vi "GetTangent(SubVI).vi"(10 "sn":string) -> (2 "output frame":string)   [LabVIEW 2012]
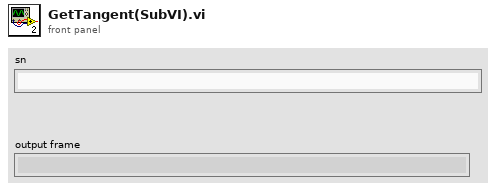
[diagram p1: front panel]
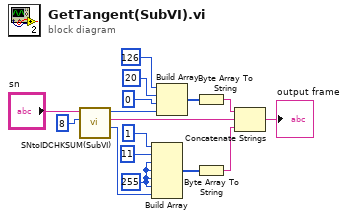
[diagram p0: block diagram]
diagram:
  w14 = u8 255
  n1 = call "SNtoIDCHKSUM(SubVI).vi"("fix cheksum"=u8 8, "input sn"="sn") -> ("output check sum"=w15:u8, "output sn"=w10:string, "output id"=w3:u8)  [unwired: 7 in]
  n2 = Build Array(u8 1, u8 11, w14, w14, w14, w14, w15) -> (w7:u8[])
  n3 = Build Array(u8 126, u8 20, u8 0, w3) -> (w8:u8[])
  n4 = Byte Array To String(unsigned byte array=w8) -> (string=w9:string)
  n5 = Byte Array To String(unsigned byte array=w7) -> (string=w11:string)
  n6 = Concatenate Strings(w9, w10, w11) -> (→"output frame":string)
